vi "cộng trừ nhân chia.vi"() -> ()   [LabVIEW 2020]
panel:
  out "chia":dbl
  out "nhan":dbl
  out "tru":dbl
  in  "stop":bool
  out "cong":dbl
  in  "Numeric 2":dbl
  in  "Numeric":dbl
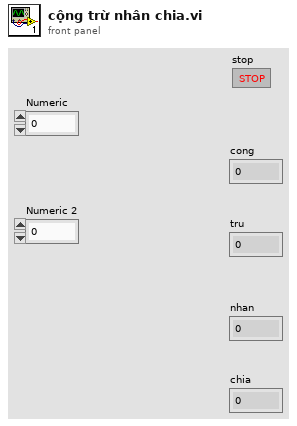
[diagram p1: front panel]
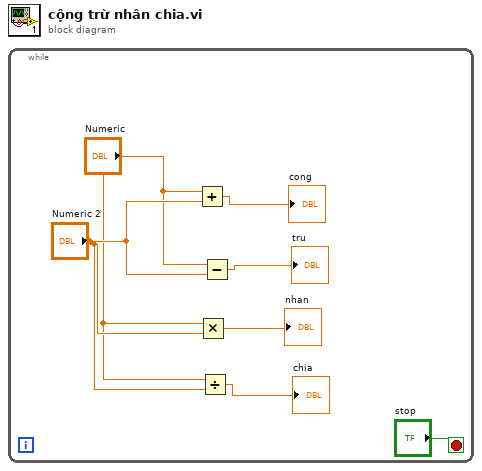
[diagram p0: block diagram]
diagram:
  n1 = while {
    stop <- "stop" stop-if-true
    n2 = Add(x="Numeric", y="Numeric 2") -> (x+y=→"cong":dbl)
    n3 = Multiply(x="Numeric", y="Numeric 2") -> (x*y=→"nhan":dbl)
    n4 = Divide(x="Numeric", y="Numeric 2") -> (x/y=→"chia":dbl)
    n5 = Subtract(x="Numeric", y="Numeric 2") -> (x-y=→"tru":dbl)
  }
